vi "FPGA Personality.vi"() -> ()   [LabVIEW 2018]
uses:
  <vilib>/rvi/Emulation/niFpgaGetClockAttributes.vi
  <vilib>/rvi/Emulation/niFpgaSctlEmulationGetInTimedLoop.vi
  <vilib>/rvi/Emulation/niFpgaEmulationReportErrorSimple.vi
  <vilib>/rvi/Emulation/niFpgaCriticalErrorInLSC.vi
  <vilib>/rvi/DataTransferAndStorage/Container/XNode/niFpgaContainer.xnode
  <vilib>/rvi/interface/RandomDataEmulation/nirviRandomDataFpgaReadWriteTemplate.vi
panel:
  out "Element":sgl
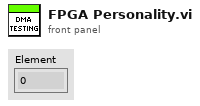
[diagram p1: front panel]
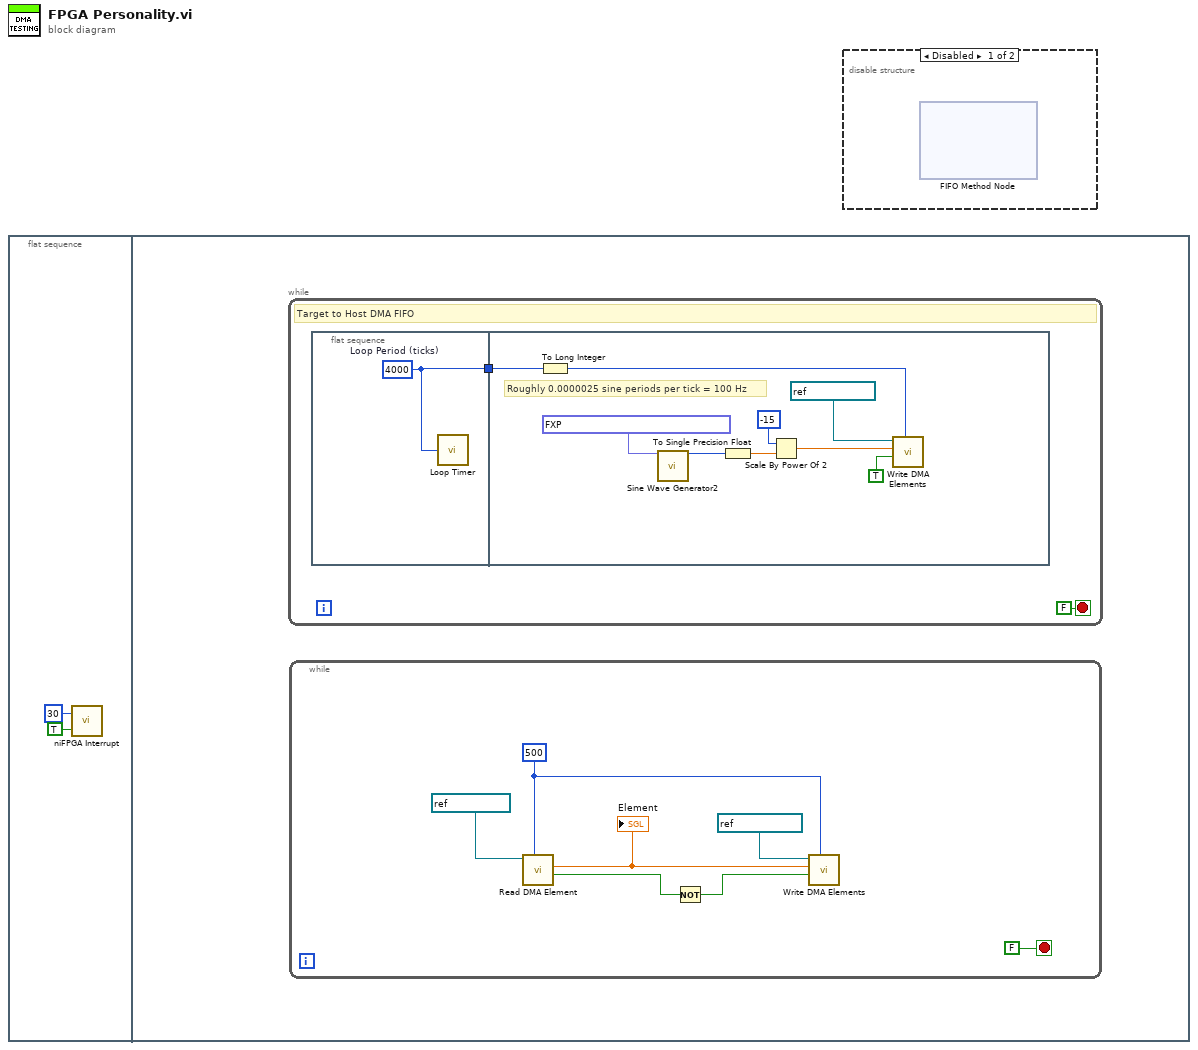
[diagram p0: block diagram]
diagram:
  n1 = flat-sequence {
    frame #0 {
      n2 = call <vilib>:"niFPGA Interrupt.vi"("Wait Until Cleared (F)"=TRUE, "IRQ Number (0)"=u8 30) -> ()  [unwired: 1 in]
    }
    frame #1 {
      n3 = while {
        stop <- FALSE stop-if-true
        # "Target to Host DMA FIFO"
        n4 = flat-sequence {
          tunnel: [w12] -> w11
          tunnel: w11 -> [w21]
          frame #0 {
            w12 = u32 4000  # Loop Period (ticks)
            n5 = call "Loop Timer"("Count(Ticks)"=w12) -> ()  [unwired: 1 out]
          }
          frame #1 {
            # "Roughly 0.0000025 sine periods per tick = 100 Hz"
            n6 = To Long Integer(number=w21) -> (32bit integer=w13:i32)
            n7 = call "Sine Wave Generator2"("frequency (periods/tick)"=fxp<+,32,0> 2.499902620911598e-06) -> ("sine out"=w18:i16)  [unwired: 14 in]
            n8 = To Single Precision Float(number=w18) -> (single precision float=w17:sgl)
            n9 = Scale By Power Of 2(n=i16 -15, x=w17) -> (x*2^n=w15:sgl)
            n10 = call "Write DMA Elements.vi"("Timeout"=w13, "isValid ?"=TRUE, "DMA Element"=w15, "FIFO Refnum in"=refnum<k21> "Outgoing1" ("FIFO In")) -> ()  [unwired: 7 in, 1 out]
          }
        }
      }
      n11 = while {
        stop <- FALSE stop-if-true
        w4 = 500 ("Timeout")
        n12 = call "Read DMA Element.vi"("Timeout"=w4, "DMA Refnum in"=refnum<k21> "Incoming" ("FIFO In")) -> ("isTimeout ?"=w7:bool, "DMA Element"=w5:sgl)  [unwired: 7 in, 1 out]
        "Element" <- w5
        n13 = Not(x=w7) -> (.not. x?=w3:bool)
        n14 = call "Write DMA Elements.vi"("Timeout"=w4, "isValid ?"=w3, "DMA Element"=w5, "FIFO Refnum in"=refnum<k21> "Outgoing2" ("FIFO In")) -> ()  [unwired: 7 in, 1 out]
      }
    }
  }
  n15 = disable-structure shown="Disabled" {
    frame Disabled {
      n16 = xnode ("FIFO Method Node")() -> ()  [unwired: 3 in, 2 out]
    }
    frame Enabled {
    }
  }
